vi "Filepather.vi"(9 "File extension":string, 10 "Filename":string, 11 "Path in":path) -> (2 "Full filepath":string, 3 "Path out":path)   [LabVIEW 2023]
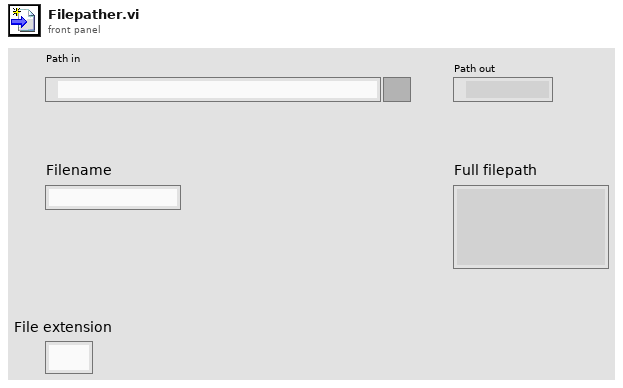
[diagram p1: front panel]
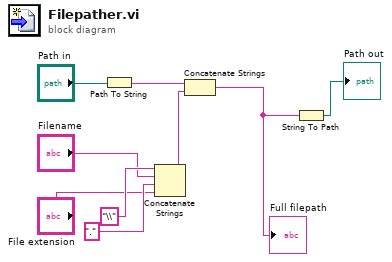
[diagram p0: block diagram]
diagram:
  n1 = Path To String(path="Path in") -> (string=w2:string)
  n2 = Concatenate Strings("\\", "Filename", ".", "File extension") -> (w1:string)
  n3 = Concatenate Strings(w2, w1) -> (w8:string)
  "Full filepath" <- w8
  n4 = String To Path(string=w8) -> (path=→"Path out":path)
